vi "Send Command.vi"(8 "error in":errorcluster, 9 "Value":variant, 10 "Command":string, 11 "PowerSupply in":refnum<class "PowerSupply.lvclass">) -> (0 "error out":errorcluster, 3 "PowerSupply out":refnum<class "PowerSupply.lvclass">)   [LabVIEW 2019, in "PowerSupply.lvlib" / "PowerSupply.lvclass"]
uses:
  Library/PowerSupply.lvclass
  C:/Users/Public/Documents/Development/builds/Engine/Engine.lvlibp/Project/Engine.lvclass
  C:/Users/Public/Documents/Development/builds/Engine/Monitored Actor.lvlibp/Monitored Actor/Monitored Actor/Monitored Actor.lvclass
  PowerSupply Messages/Write Active Channel Msg/Write Active Channel Msg.lvclass/Write Active Channel Msg.ctl
  PowerSupply Messages/Write Limit Current Msg/Write Limit Current Msg.lvclass/Write Limit Current Msg.ctl
  PowerSupply Messages/Write Ramp Current Msg/Write Ramp Current Msg.lvclass/Write Ramp Current Msg.ctl
  PowerSupply Messages/Write Current Msg/Write Current Msg.lvclass/Write Current Msg.ctl
  PowerSupply Messages/Write Current_Share Msg/Write Current_Share Msg.lvclass/Write Current_Share Msg.ctl
  PowerSupply Messages/Write Interlock_Enable Msg/Write Interlock_Enable Msg.lvclass/Write Interlock_Enable Msg.ctl
  PowerSupply Messages/Write OCP_Mode Msg/Write OCP_Mode Msg.lvclass/Write OCP_Mode Msg.ctl
  PowerSupply Messages/Write OCP_Enable Msg/Write OCP_Enable Msg.lvclass/Write OCP_Enable Msg.ctl
  PowerSupply Messages/Write Output_Enable Msg/Write Output_Enable Msg.lvclass/Write Output_Enable Msg.ctl
  PowerSupply Messages/Write OVP_Enable Msg/Write OVP_Enable Msg.lvclass/Write OVP_Enable Msg.ctl
  PowerSupply Messages/Write Sense_Point Msg/Write Sense_Point Msg.lvclass/Write Sense_Point Msg.ctl
  PowerSupply Messages/Write Limit Volt Msg/Write Limit Volt Msg.lvclass/Write Limit Volt Msg.ctl
  PowerSupply Messages/Write Ramp Volt Msg/Write Ramp Volt Msg.lvclass/Write Ramp Volt Msg.ctl
  PowerSupply Messages/Write Voltage Msg/Write Voltage Msg.lvclass/Write Voltage Msg.ctl
  builds/Engine/Engine.lvlibp/Accessors/Read Self Q.vi
  builds/Engine/Monitored Actor.lvlibp/Monitored Actor/Monitored Actor/Read Actor Label.vi
  builds/Engine/Actor Framework.lvlibp/1abvi3w/vi.lib/ActorFramework/Message Enqueuer/Enqueue.vi
  <vilib>/Utility/error.llb/Error Cluster From Error Code.vi
  builds/Engine/Actor Framework.lvlibp/1abvi3w/vi.lib/ActorFramework/Message Enqueuer/Message Enqueuer.lvclass
  PowerSupply Messages/Write Active Channel Msg/Write Active Channel Msg.lvclass
  PowerSupply Messages/Write Limit Current Msg/Write Limit Current Msg.lvclass
  PowerSupply Messages/Write Ramp Current Msg/Write Ramp Current Msg.lvclass
  PowerSupply Messages/Write Current Msg/Write Current Msg.lvclass
  PowerSupply Messages/Write Current_Share Msg/Write Current_Share Msg.lvclass
  PowerSupply Messages/Write Interlock_Enable Msg/Write Interlock_Enable Msg.lvclass
  PowerSupply Messages/Write OCP_Mode Msg/Write OCP_Mode Msg.lvclass
  PowerSupply Messages/Write OCP_Enable Msg/Write OCP_Enable Msg.lvclass
  PowerSupply Messages/Write Output_Enable Msg/Write Output_Enable Msg.lvclass
  PowerSupply Messages/Write OVP_Enable Msg/Write OVP_Enable Msg.lvclass
  PowerSupply Messages/Reset Supply Msg/Reset Supply Msg.lvclass
  PowerSupply Messages/Write Sense_Point Msg/Write Sense_Point Msg.lvclass
  PowerSupply Messages/Synch From Supply Msg/Synch From Supply Msg.lvclass
  PowerSupply Messages/Write Limit Volt Msg/Write Limit Volt Msg.lvclass
  PowerSupply Messages/Write Ramp Volt Msg/Write Ramp Volt Msg.lvclass
  PowerSupply Messages/Write Voltage Msg/Write Voltage Msg.lvclass
  <vilib>/ErrorRing/Error Ring.xnode
  builds/Engine/Engine.lvlibp/Project/Engine.lvclass
  builds/Instruments/Instruments.lvlibp/Instruments Messages/Power Off Msg/Power Off Msg.lvclass
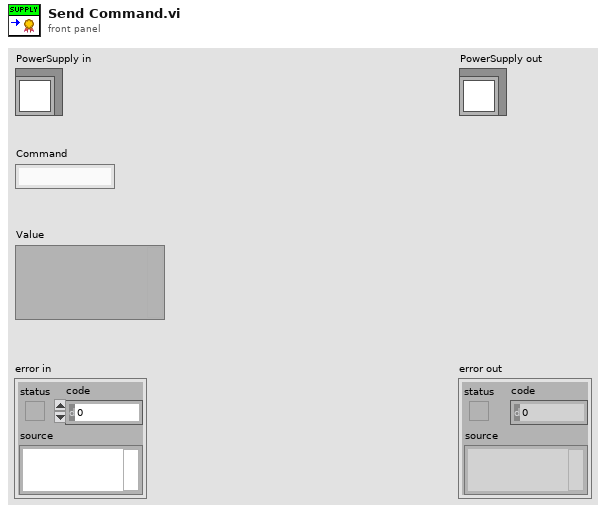
[diagram p1: front panel]
types:
  T1 = typedef "PowerSupply.lvlib/PowerSupply.lvclass/OCP Mode.ctl" = enum16{"Shutdown", "Foldback"}
  T2 = typedef "PowerSupply.lvlib/PowerSupply.lvclass/Sense Point.ctl" = enum16{"Local", "Remote"}
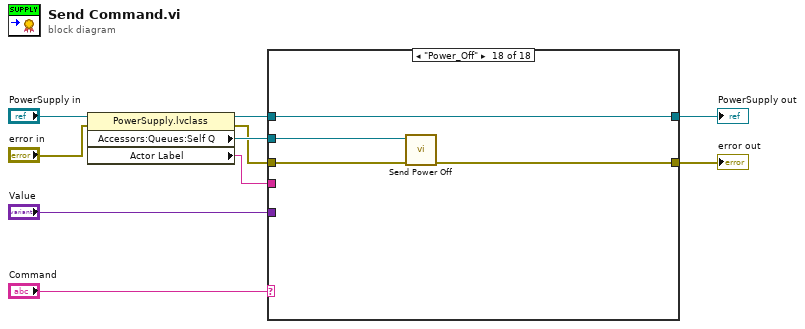
[diagram p0: block diagram]
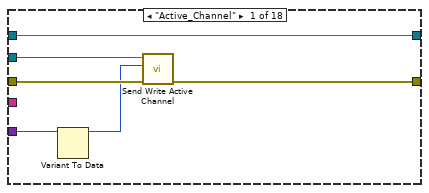
[diagram p2: hidden frame]
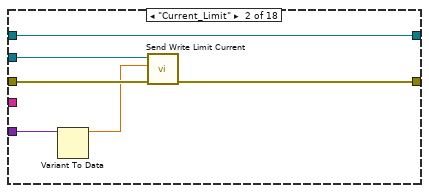
[diagram p3: hidden frame]
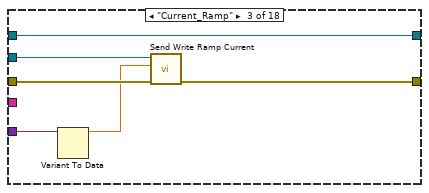
[diagram p4: hidden frame]
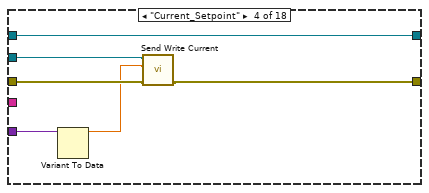
[diagram p5: hidden frame]
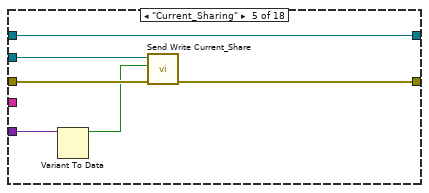
[diagram p6: hidden frame]
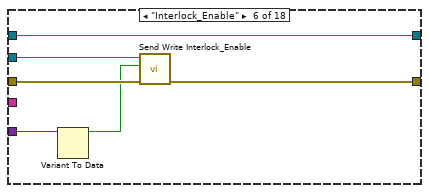
[diagram p7: hidden frame]
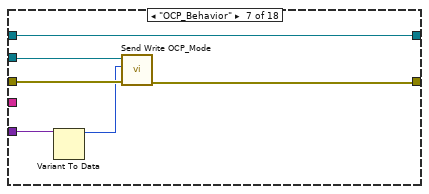
[diagram p8: hidden frame]
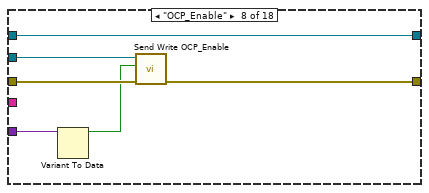
[diagram p9: hidden frame]
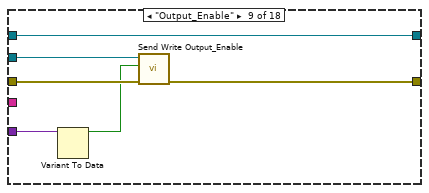
[diagram p10: hidden frame]
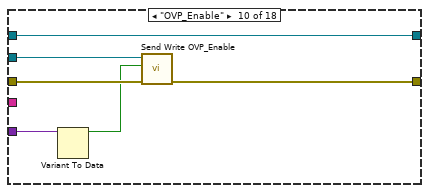
[diagram p11: hidden frame]
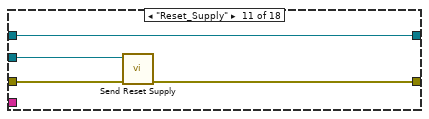
[diagram p12: hidden frame]
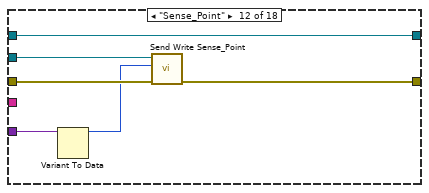
[diagram p13: hidden frame]
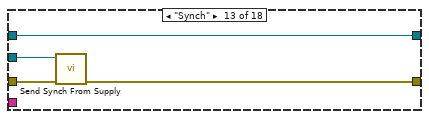
[diagram p14: hidden frame]
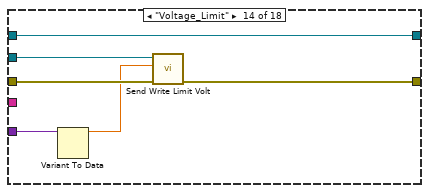
[diagram p15: hidden frame]
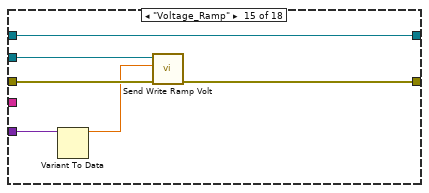
[diagram p16: hidden frame]
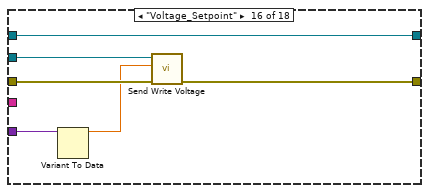
[diagram p17: hidden frame]
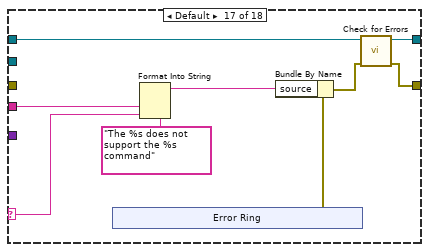
[diagram p18: hidden frame]
diagram:
  n1 = property class="PowerSupply.lvclass"(reference="PowerSupply in", error in="error in") -> (reference out=w6:refnum<class "PowerSupply.lvclass">, error out=w3:errorcluster, "Accessors:Queues:Self Q"=w4:refnum<class "Message Enqueuer.lvclass">, "Actor Label"=w1:string)
  n2 = case shown="\"Power_Off\"" "Command" {
    selector: "Command" -> [_ _ _ _ _ _ _ _ _ _ _ _ _ _ _ _ w103 _]
    tunnel: "Value" -> [w12 w21 w27 w33 w39 w45 w51 w57 w63 w69 _ w79 _ w89 w95 w101 _ _]
    tunnel: w6 -> [w16 w22 w28 w34 w40 w46 w52 w58 w64 w70 w74 w80 w84 w90 w96 w102 w111 w119]
    tunnel: [w16 w22 w28 w34 w40 w46 w52 w58 w64 w70 w74 w80 w84 w90 w96 w102 w110 w119] -> w5
    tunnel: w4 -> [w14 w18 w24 w30 w37 w41 w50 w54 w60 w66 w73 w75 w82 w87 w92 w98 _ w118]
    tunnel: w3 -> [w15 w20 w26 w32 w38 w44 w49 w56 w62 w68 w72 w78 w83 w88 w94 w100 _ w117]
    tunnel: [w13 w19 w25 w29 w35 w43 w48 w55 w61 w67 w71 w77 w81 w85 w93 w99 w109 w116] -> w2
    tunnel: w1 -> [_ _ _ _ _ _ _ _ _ _ _ _ _ _ _ _ w107 _]
    frame "Active_Channel" {
      n3 = Variant To Data(Variant=w12) -> (data=w11:u32)  [unwired: 2 in, 1 out]
      n4 = call "Send Write Active Channel.vi"("error in (no error)"=w15, "Active Channel"=w11, "Message Enqueuer"=w14) -> ("error out"=w13:errorcluster)  [unwired: 7 in, 1 out]
    }
    frame "Current_Limit" {
      n5 = Variant To Data(Variant=w21) -> (data=w17:dbl)  [unwired: 2 in, 1 out]
      n6 = call "Send Write Limit Current.vi"("error in (no error)"=w20, "OverCurrent_Protect"=w17, "Message Enqueuer"=w18) -> ("error out"=w19:errorcluster)  [unwired: 7 in, 1 out]
    }
    frame "Current_Ramp" {
      n7 = Variant To Data(Variant=w27) -> (data=w23:dbl)  [unwired: 2 in, 1 out]
      n8 = call "Send Write Ramp Current.vi"("error in (no error)"=w26, "Current_Ramp"=w23, "Message Enqueuer"=w24) -> ("error out"=w25:errorcluster)  [unwired: 7 in, 1 out]
    }
    frame "Current_Setpoint" {
      n9 = Variant To Data(Variant=w33) -> (data=w31:dbl)  [unwired: 2 in, 1 out]
      n10 = call "Send Write Current.vi"("error in (no error)"=w32, "Current"=w31, "Message Enqueuer"=w30) -> ("error out"=w29:errorcluster)  [unwired: 7 in, 1 out]
    }
    frame "Current_Sharing" {
      n11 = Variant To Data(Variant=w39) -> (data=w36:bool)  [unwired: 2 in, 1 out]
      n12 = call "Send Write Current_Share.vi"("error in (no error)"=w38, "Current_Sharing"=w36, "Message Enqueuer"=w37) -> ("error out"=w35:errorcluster)  [unwired: 7 in, 1 out]
    }
    frame "Interlock_Enable" {
      n13 = Variant To Data(Variant=w45) -> (data=w42:bool)  [unwired: 2 in, 1 out]
      n14 = call "Send Write Interlock_Enable.vi"("error in (no error)"=w44, "INTLK_Enable"=w42, "Message Enqueuer"=w41) -> ("error out"=w43:errorcluster)  [unwired: 7 in, 1 out]
    }
    frame "OCP_Behavior" {
      n15 = Variant To Data(Variant=w51) -> (data=w47:T1)  [unwired: 2 in, 1 out]
      n16 = call "Send Write OCP_Mode.vi"("error in (no error)"=w49, "OCP Mode"=w47, "Message Enqueuer"=w50) -> ("error out"=w48:errorcluster)  [unwired: 7 in, 1 out]
    }
    frame "OCP_Enable" {
      n17 = Variant To Data(Variant=w57) -> (data=w53:bool)  [unwired: 2 in, 1 out]
      n18 = call "Send Write OCP_Enable.vi"("error in (no error)"=w56, "OCP_Enable"=w53, "Message Enqueuer"=w54) -> ("error out"=w55:errorcluster)  [unwired: 7 in, 1 out]
    }
    frame "Output_Enable" {
      n19 = Variant To Data(Variant=w63) -> (data=w59:bool)  [unwired: 2 in, 1 out]
      n20 = call "Send Write Output_Enable.vi"("error in (no error)"=w62, "Output_Enable"=w59, "Message Enqueuer"=w60) -> ("error out"=w61:errorcluster)  [unwired: 7 in, 1 out]
    }
    frame "OVP_Enable" {
      n21 = Variant To Data(Variant=w69) -> (data=w65:bool)  [unwired: 2 in, 1 out]
      n22 = call "Send Write OVP_Enable.vi"("error in (no error)"=w68, "OVP_Enable"=w65, "Message Enqueuer"=w66) -> ("error out"=w67:errorcluster)  [unwired: 7 in, 1 out]
    }
    frame "Reset_Supply" {
      n23 = call "Send Reset Supply.vi"("error in (no error)"=w72, "Message Enqueuer"=w73) -> ("error out"=w71:errorcluster)  [unwired: 8 in, 1 out]
    }
    frame "Sense_Point" {
      n24 = Variant To Data(Variant=w79) -> (data=w76:T2)  [unwired: 2 in, 1 out]
      n25 = call "Send Write Sense_Point.vi"("error in (no error)"=w78, "Sense Point"=w76, "Message Enqueuer"=w75) -> ("error out"=w77:errorcluster)  [unwired: 7 in, 1 out]
    }
    frame "Synch" {
      n26 = call "Send Synch From Supply.vi"("error in (no error)"=w83, "Message Enqueuer"=w82) -> ("error out"=w81:errorcluster)  [unwired: 8 in, 1 out]
    }
    frame "Voltage_Limit" {
      n27 = Variant To Data(Variant=w89) -> (data=w86:dbl)  [unwired: 2 in, 1 out]
      n28 = call "Send Write Limit Volt.vi"("error in (no error)"=w88, "OverVolt_Protect"=w86, "Message Enqueuer"=w87) -> ("error out"=w85:errorcluster)  [unwired: 7 in, 1 out]
    }
    frame "Voltage_Ramp" {
      n29 = Variant To Data(Variant=w95) -> (data=w91:dbl)  [unwired: 2 in, 1 out]
      n30 = call "Send Write Ramp Volt.vi"("error in (no error)"=w94, "Voltage_Ramp"=w91, "Message Enqueuer"=w92) -> ("error out"=w93:errorcluster)  [unwired: 7 in, 1 out]
    }
    frame "Voltage_Setpoint" {
      n31 = Variant To Data(Variant=w101) -> (data=w97:dbl)  [unwired: 2 in, 1 out]
      n32 = call "Send Write Voltage.vi"("error in (no error)"=w100, "Voltage"=w97, "Message Enqueuer"=w98) -> ("error out"=w99:errorcluster)  [unwired: 7 in, 1 out]
    }
    frame Default {
      n33 = xnode "Error Ring"() -> ("error out"=w108:errorcluster)
      n34 = Format Into String(format string="The %s does not support the %s command", w107, w103) -> (resulting string=w106:string)  [unwired: 2 in, 1 out]
      n35 = Bundle By Name(cluster=w108, "source"=w106) -> (w105:errorcluster)
      n36 = call "Check for Errors.vi"("error in"=w105, "Engine in"=w111) -> ("error out"=w109:errorcluster, "Engine out"=w110:refnum<class "PowerSupply.lvclass">)  [unwired: 8 in]
    }
    frame "Power_Off" {
      n37 = call "Send Power Off.vi"("error in (no error)"=w117, "Message Enqueuer"=w118) -> ("error out"=w116:errorcluster)  [unwired: 8 in, 1 out]
    }
  }
  "error out" <- w2
  "PowerSupply out" <- w5
